vi "Ptogramacion practica de examen lectura.vi"() -> ()   [LabVIEW 2011]
panel:
  out "Array":T1(array[cluster]) {"diesel" scale=0.0..500.0; "Gasolina r" scale=0.0..500.0; "Gasolina S" scale=0.0..500.0}
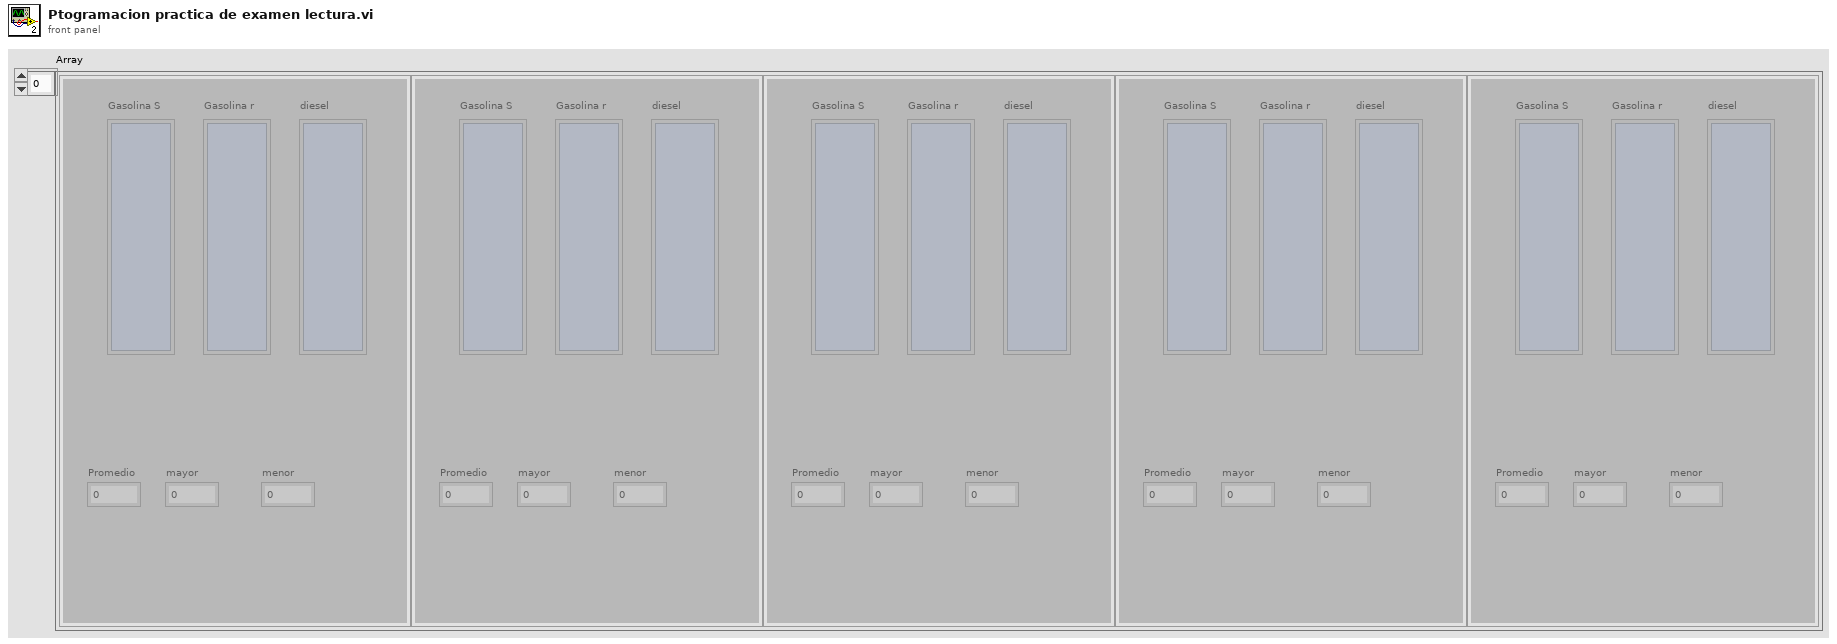
[diagram p1: front panel]
types:
  T1 = cluster{"Gasolina S":i32, "Gasolina r":i32, "diesel":i32, "Promedio":dbl, "mayor":dbl, "menor":dbl}[]
  T2 = enum16{"open", "replace", "create", "open or create", "replace or create", "replace or create with confirmation"}
  T3 = cluster{"Gasolina S":i32, "Gasolina r":i32, "diesel":i32, "Promedio":dbl, "mayor":dbl, "menor":dbl}
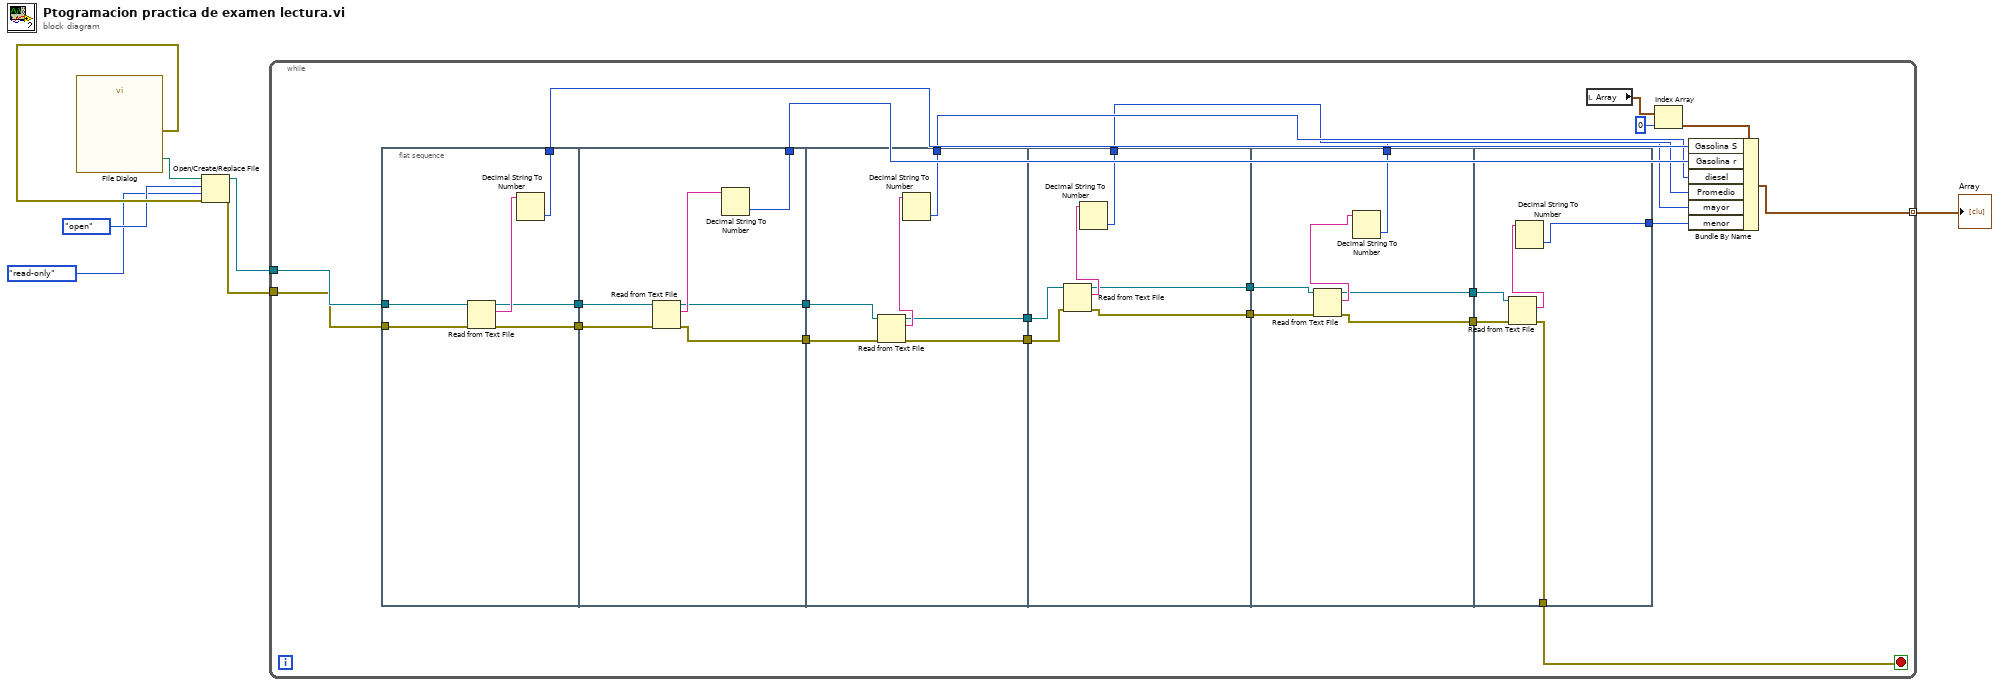
[diagram p0: block diagram]
diagram:
  n1 = call "File Dialog"() -> ("selected path"=w7:path, "error out"=w6:errorcluster)  [unwired: 12 in, 2 out]
  n2 = Open/Create/Replace File(file path (use dialog)=w7, error in=w6, operation (0:open)=T2."open", access (0:read/write)=enum16{"read/write", "read-only", "write-only"}."read-only") -> (refnum out=w3:refnum<file>, error out=w2:errorcluster)  [unwired: 2 in, 1 out]
  n3 = while {
    tunnel: w3 -> [w30]
    tunnel: w2 -> [w29]
    tunnel: [w8] -> w1 mode=indexing
    stop <- w9 stop-if-true
    n4 = flat-sequence {
      tunnel: w30 -> [w36]
      tunnel: w29 -> [w35]
      tunnel: [w33] -> w25
      tunnel: [w32] -> w24
      tunnel: [w31] -> w23
      tunnel: w24 -> [w42]
      tunnel: w23 -> [w41]
      tunnel: [w39] -> w22
      tunnel: [w38] -> w21
      tunnel: [w37] -> w20
      tunnel: w21 -> [w48]
      tunnel: w20 -> [w47]
      tunnel: [w45] -> w19
      tunnel: [w44] -> w18
      tunnel: [w43] -> w17
      tunnel: w18 -> [w54]
      tunnel: w17 -> [w53]
      tunnel: [w51] -> w16
      tunnel: [w50] -> w15
      tunnel: [w49] -> w14
      tunnel: w15 -> [w60]
      tunnel: w14 -> [w59]
      tunnel: [w57] -> w13
      tunnel: [w56] -> w12
      tunnel: [w55] -> w11
      tunnel: w12 -> [w65]
      tunnel: w11 -> [w64]
      tunnel: [w62] -> w10
      tunnel: [w61] -> w9
      frame #0 {
        n5 = Read from Text File(file (use dialog)=w36, error in=w35) -> (refnum out=w32:refnum<file>, text=w34:string, error out=w31:errorcluster)  [unwired: 2 in, 1 out]
        n6 = Decimal String To Number(string=w34) -> (number=w33:i32)  [unwired: 2 in, 1 out]
      }
      frame #1 {
        n7 = Read from Text File(file (use dialog)=w42, error in=w41) -> (refnum out=w38:refnum<file>, text=w40:string, error out=w37:errorcluster)  [unwired: 2 in, 1 out]
        n8 = Decimal String To Number(string=w40) -> (number=w39:i32)  [unwired: 2 in, 1 out]
      }
      frame #2 {
        n9 = Read from Text File(file (use dialog)=w48, error in=w47) -> (refnum out=w44:refnum<file>, text=w46:string, error out=w43:errorcluster)  [unwired: 2 in, 1 out]
        n10 = Decimal String To Number(string=w46) -> (number=w45:i32)  [unwired: 2 in, 1 out]
      }
      frame #3 {
        n11 = Read from Text File(file (use dialog)=w54, error in=w53) -> (refnum out=w50:refnum<file>, text=w52:string, error out=w49:errorcluster)  [unwired: 2 in, 1 out]
        n12 = Decimal String To Number(string=w52) -> (number=w51:i32)  [unwired: 2 in, 1 out]
      }
      frame #4 {
        n13 = Read from Text File(file (use dialog)=w60, error in=w59) -> (refnum out=w56:refnum<file>, text=w58:string, error out=w55:errorcluster)  [unwired: 2 in, 1 out]
        n14 = Decimal String To Number(string=w58) -> (number=w57:i32)  [unwired: 2 in, 1 out]
      }
      frame #5 {
        n15 = Read from Text File(file (use dialog)=w65, error in=w64) -> (text=w63:string, error out=w61:errorcluster)  [unwired: 2 in, 2 out]
        n16 = Decimal String To Number(string=w63) -> (number=w62:i32)  [unwired: 2 in, 1 out]
      }
    }
    n17 = local read "Array"() -> (w28:T1)
    n18 = Index Array(array=w28, index=0) -> (element=w26:T3)
    n19 = Bundle By Name(cluster=w26, "Gasolina S"=w25, "Gasolina r"=w22, "diesel"=w19, "Promedio"=w16, "mayor"=w13, "menor"=w10) -> (w8:T3)
  }
  "Array" <- w1
